vi "Angle Measurement.vi"() -> ()   [LabVIEW 2020]
panel:
  out "Numeric 2":dbl
  in  "stop":bool
  out "Numeric":dbl
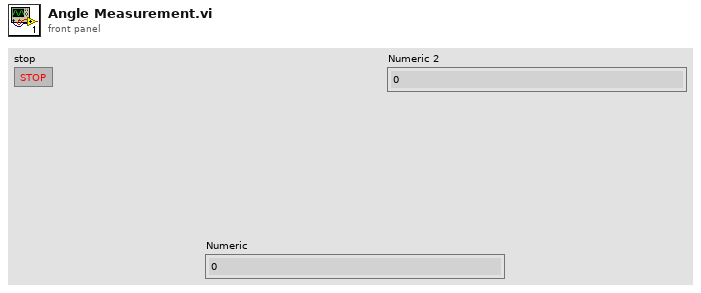
[diagram p1: front panel]
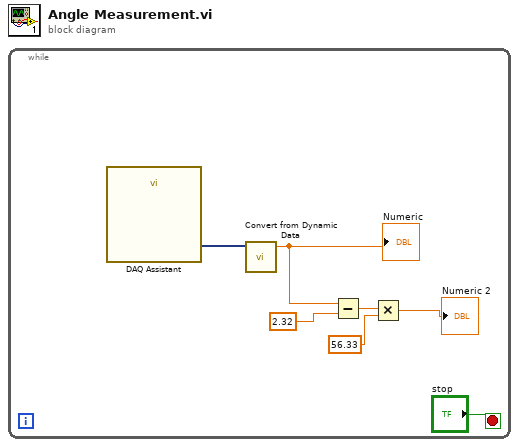
[diagram p0: block diagram]
diagram:
  n1 = while {
    stop <- "stop" stop-if-true
    n2 = call "DAQ Assistant"() -> ("data"=w7:dynamicdata)  [unwired: 17 in, 2 out]
    n3 = call "Convert from Dynamic Data"("Dynamic Data Type"=w7) -> ("Scalar"=w5:dbl)  [unwired: 3 in]
    "Numeric" <- w5
    n4 = Subtract(x=w5, y=2.32) -> (x-y=w3:dbl)
    n5 = Multiply(x=w3, y=56.33) -> (x*y=→"Numeric 2":dbl)
  }
